vi "MarksScored_ForStructureQn(SubVI).vi"(8 "TotalMarks?":string, 9 "+?Marks":dbl, 10 "Marks/QnPartsCorrect":dbl=0.5, 11 "No.ofMatchedKeywords":i32[](array[numeric])) -> (0 "MarksScored":string)   [LabVIEW 2013]
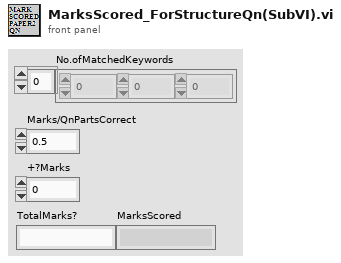
[diagram p1: front panel]
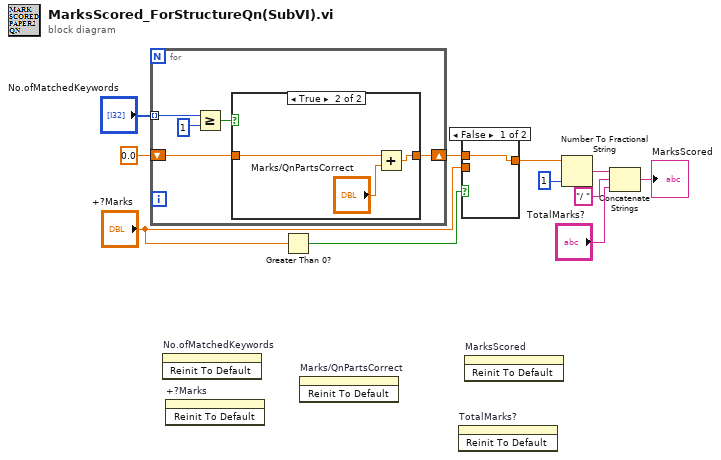
[diagram p0: block diagram]
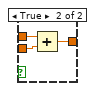
[diagram p2: hidden frame]
diagram:
  n1 = for {
    tunnel: "No.ofMatchedKeywords" -> [w15] mode=indexing
    shift-right: [w12] -> w6
    shift-left: 0.0 -> [w13]
    n2 = Greater Or Equal?(x=w15, y=1) -> (x >= y?=w14:bool)
    n3 = case shown="True" w14 {
      tunnel: w13 -> [w17 w20]
      tunnel: [w17 w18] -> w12
      frame False {
      }
      frame True {
        n4 = Add(x=w20, y="Marks/QnPartsCorrect") -> (x+y=w18:dbl)
      }
    }
  }
  n5 = invoke on="No.ofMatchedKeywords" class="Arr (strict)" method="Reinit To Default"() -> ()  [unwired: 3 in, 3 out]
  n6 = invoke on="+?Marks" class="DigNum (strict)" method="Reinit To Default"() -> ()  [unwired: 3 in, 3 out]
  n7 = Greater Than 0?(x="+?Marks") -> (x > 0?=w4:bool)
  n8 = invoke on="Marks/QnPartsCorrect" class="DigNum (strict)" method="Reinit To Default"() -> ()  [unwired: 3 in, 3 out]
  n9 = invoke on="TotalMarks?" class="Str" method="Reinit To Default"() -> ()  [unwired: 3 in, 3 out]
  n10 = case shown="False" w4 {
    tunnel: [w21 w24] -> w7
    tunnel: w6 -> [w21 w23]
    tunnel: "+?Marks" -> [_ w22]
    frame False {
    }
    frame True {
      n11 = Add(x=w23, y=w22) -> (x+y=w24:dbl)
    }
  }
  n12 = invoke on="MarksScored" class="Str" method="Reinit To Default"() -> ()  [unwired: 3 in, 3 out]
  n13 = Number To Fractional String(number=w7, precision (6)=i16 1) -> (F-format string=w2:string)  [unwired: 2 in]
  n14 = Concatenate Strings(w2, "/ " ("string"), "TotalMarks?") -> (→"MarksScored":string)
